vi "Read ADU Packet.vi"(8 "error in":errorcluster, 10 "protocol layer":refnum<class "Network Protocol.lvclass">, 11 "IP transmission data unit in":refnum<class "IP Data Unit.lvclass">) -> (0 "error out":errorcluster, 1 "modbus data unit":refnum<class "Modbus Data Unit.lvclass">, 2 "protocol layer out":refnum<class "Network Protocol.lvclass">, 3 "IP transmission data unit out":refnum<class "IP Data Unit.lvclass">, 5 "PDU Valid?":bool)   [LabVIEW 2013, in "IP Data Unit.lvclass"]
doc: "This uses the protocol layer to read a modbus packet off of the bus, wrapped in the IP transmission data unit."
uses:
  IP Data Unit.lvclass
  Modbus Data Unit/Modbus Data Unit.lvclass
  Network Protocol/Network Protocol.lvclass
  Transmission Data Unit.lvclass/Transmission Data Unit.ctl
  IP Data Unit.lvclass/IP Data Unit.ctl
  Modbus Data Unit/Modbus Data Unit.lvclass/Modbus Data Unit.ctl
  Modbus Data Unit/Unflatten to PDU.vi
  <vilib>/ErrorRing/Error Ring.xnode
  Transmission Data Unit.lvclass
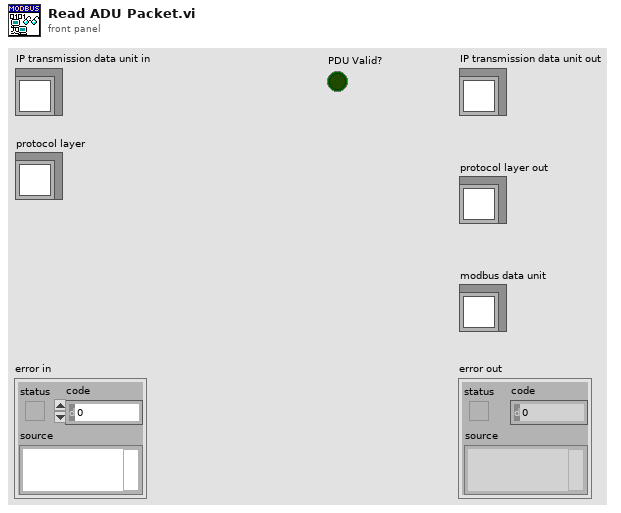
[diagram p1: front panel]
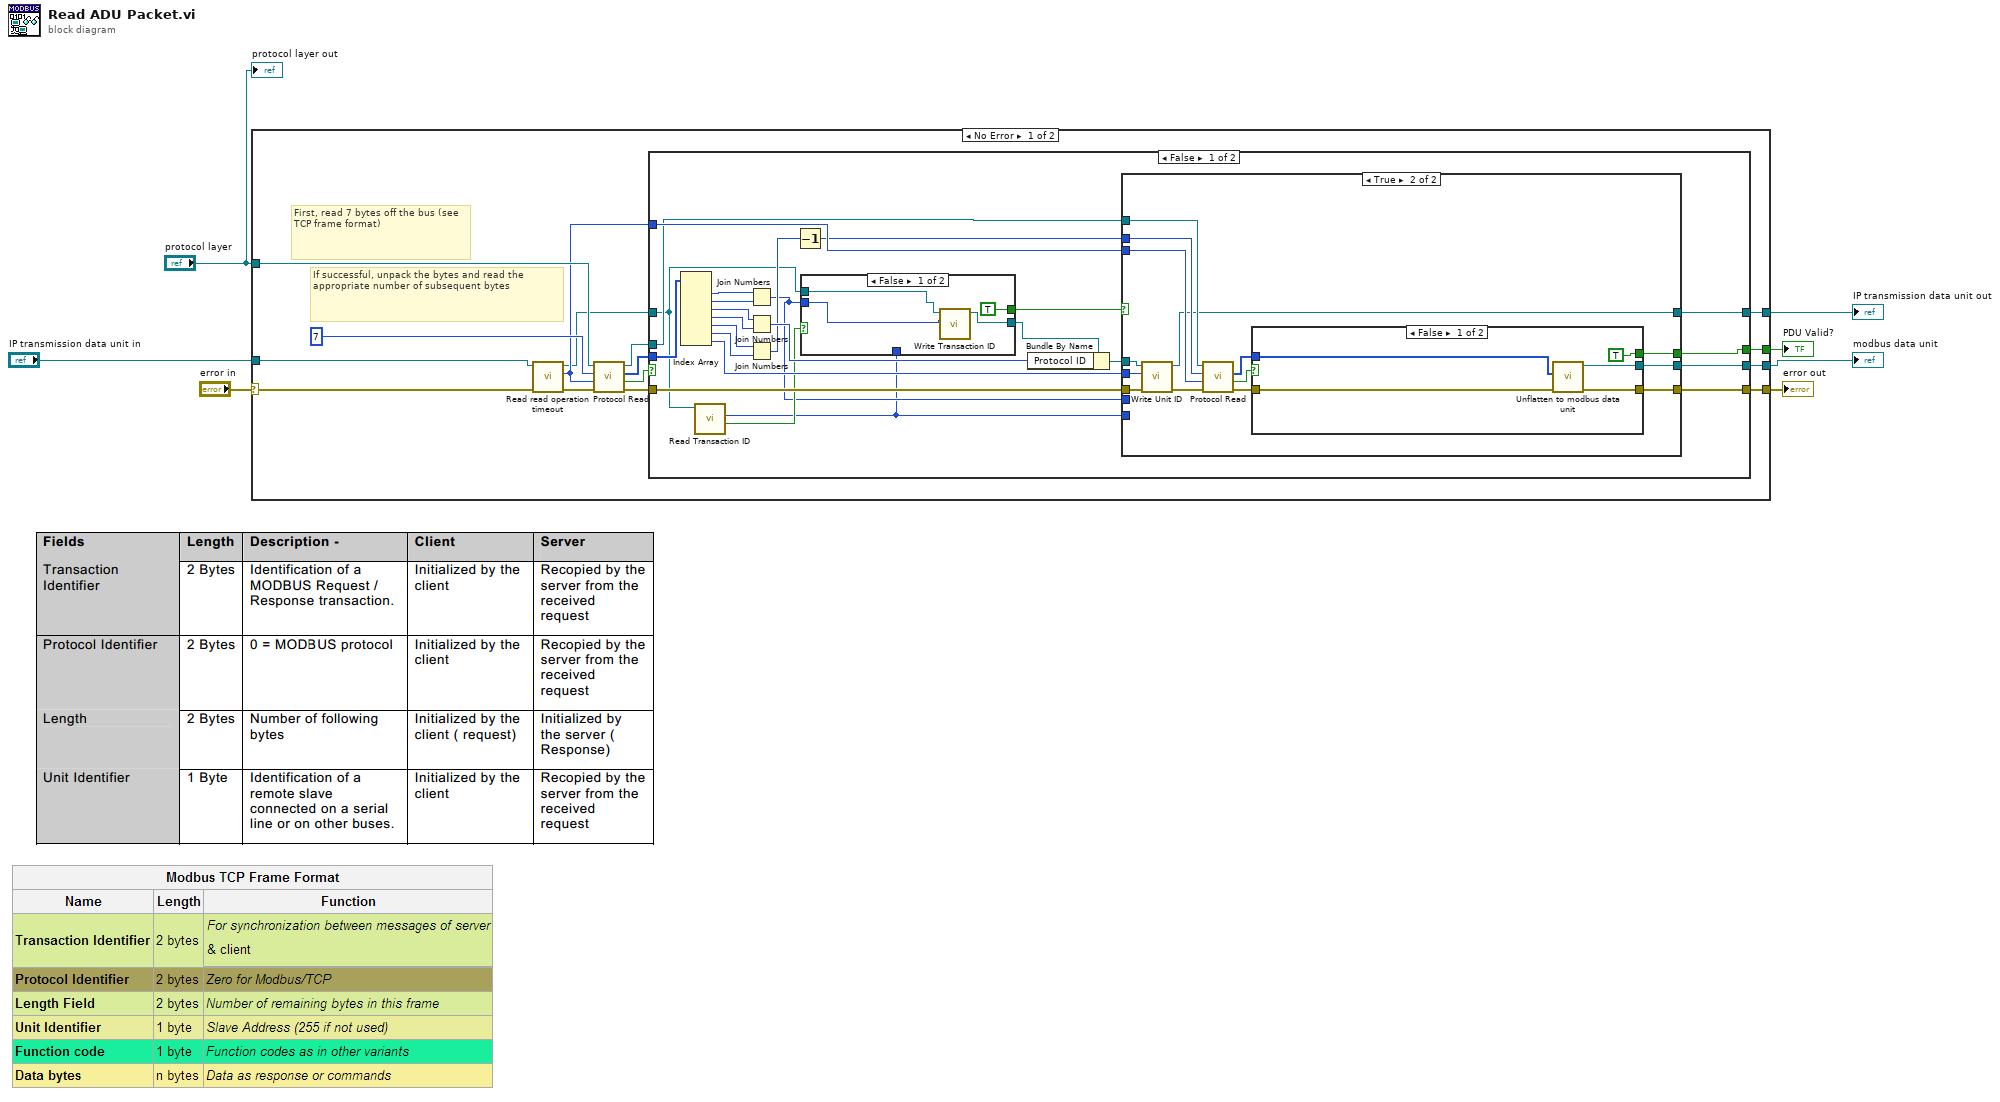
[diagram p0: block diagram]
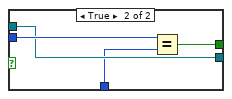
[diagram p2: hidden frame]
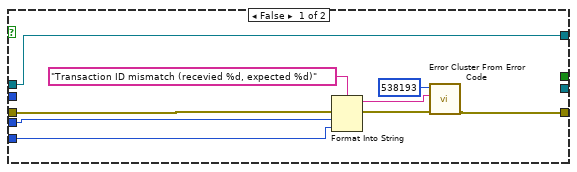
[diagram p3: hidden frame]
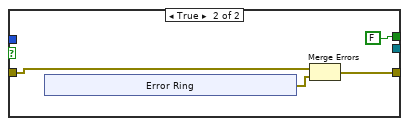
[diagram p4: hidden frame]
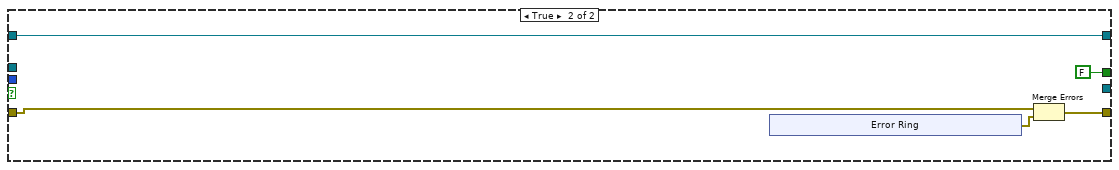
[diagram p5: hidden frame]
diagram:
  n1 = case shown="No Error" "error in" {
    selector: "error in" -> [w10 w102]
    tunnel: [w16 w102] -> w6
    tunnel: "IP transmission data unit in" -> [w12 w101]
    tunnel: [w19 w101] -> w4
    tunnel: "protocol layer" -> [w22 _]
    tunnel: [w15 _] -> w3
    tunnel: [w8 _] -> w1
    frame No Error {
      # "If successful, unpack the bytes and read the appropriate number of subsequent bytes"
      # "First, read 7 bytes off the bus (see TCP frame format)"
      n2 = call "Read read operation timeout.vi"("error in (no error)"=w10, "transmission data unit in"=w12) -> ("error out"=w9:errorcluster, "read operation timeout"=w13:i32, "transmission data unit out"=w11:refnum<class "IP Data Unit.lvclass">)  [unwired: 7 in]
      n3 = call-dynamic "Protocol Read.vi"("error in"=w9, "timeout"=w13, "bytes to read"=7 ("Bytes to Read"), "protocol layer in"=w22) -> ("error out"=w17:errorcluster, "timed out?"=w14:bool, "data"=w20:u8[], "protocol layer out"=w18:refnum<class "Network Protocol.lvclass">)  [unwired: 4 in]
      n4 = case shown="False" w14 {
        tunnel: w20 -> [w47 _]
        tunnel: w11 -> [w26 w96]
        tunnel: [w33 w96] -> w19
        tunnel: w18 -> [w29 _]
        tunnel: w13 -> [w38 _]
        tunnel: w17 -> [w27 w93]
        tunnel: [w36 w94] -> w16
        tunnel: [w35 _] -> w15
        tunnel: [w31 FALSE] -> w8
        frame False {
          n5 = Index Array(array=w47) -> (element #1=w45:u8, element #2=w46:u8, element #3=w44:u8, element #4=w43:u8, element #5=w40:u8, element #6=w41:u8, element #7=w32:u8)  [unwired: 7 in]
          n6 = call "Read Transaction ID.vi"("IP Data Unit in"=w26) -> ("Transaction ID set?"=w25:bool, "Transaction ID"=w23:u16)  [unwired: 8 in, 1 out]
          n7 = Join Numbers(hi=w45, lo=w46) -> ((hi.lo)=w24:u16)
          n8 = Join Numbers(hi=w44, lo=w43) -> ((hi.lo)=w42:u16)
          n9 = Join Numbers(hi=w40, lo=w41) -> ((hi.lo)=w39:u16)
          n10 = Decrement(x=w39) -> (x-1=w37:u16)
          n11 = case shown="False" w25 {
            tunnel: w26 -> [w50 w53]
            tunnel: w24 -> [w48 w55]
            tunnel: [TRUE w54] -> w30
            tunnel: [w49 w53] -> w28
            tunnel: w23 -> [_ w52]
            frame False {
              n12 = call "Write Transaction ID.vi"("Transaction ID"=w48, "IP Data Unit in"=w50) -> ("IP Data Unit out"=w49:refnum<class "IP Data Unit.lvclass">)  [unwired: 9 in]
            }
            frame True {
              n13 = Equal?(x=w55, y=w52) -> (x = y?=w54:bool)
            }
          }
          n14 = Bundle By Name(cluster=w28, "Protocol ID"=w42) -> (w34:refnum<class "IP Data Unit.lvclass">)
          n15 = case shown="True" w30 {
            tunnel: w29 -> [_ w78]
            tunnel: w38 -> [_ w77]
            tunnel: w37 -> [_ w76]
            tunnel: [w63 w74] -> w36
            tunnel: [_ w73] -> w35
            tunnel: w34 -> [w64 w70]
            tunnel: [w64 w69] -> w33
            tunnel: w27 -> [w61 w67]
            tunnel: w32 -> [_ w66]
            tunnel: [_ w65] -> w31
            tunnel: w24 -> [w57 _]
            tunnel: w23 -> [w56 _]
            frame False {
              n16 = Format Into String(format string="Transaction ID mismatch (recevied %d, expected %d)", error in=w61, w57, w56) -> (resulting string=w59:string, error out=w60:errorcluster)  [unwired: 1 in]
              n17 = call <vilib>:"Error Cluster From Error Code.vi"("error in (no error)"=w60, "error message (\"\")"=w59, "error code (0)"=538193) -> ("error out"=w63:errorcluster)  [unwired: 6 in]
            }
            frame True {
              n18 = call "Write Unit ID.vi"("error in"=w67, "unit ID"=w66, "transmission data unit in"=w70) -> ("error out"=w68:errorcluster, "transmission data unit out"=w69:refnum<class "IP Data Unit.lvclass">)  [unwired: 7 in]
              n19 = call-dynamic "Protocol Read.vi"("error in"=w68, "timeout"=w77, "bytes to read"=w76, "protocol layer in"=w78) -> ("error out"=w75:errorcluster, "timed out?"=w71:bool, "data"=w72:u8[])  [unwired: 4 in, 1 out]
              n20 = case shown="False" w71 {
                tunnel: w75 -> [w83 w86]
                tunnel: [w82 w87] -> w74
                tunnel: [w81 _] -> w73
                tunnel: w72 -> [w80 _]
                tunnel: [TRUE FALSE] -> w65
                frame False {
                  n21 = call "Unflatten to modbus data unit.vi"("error in"=w83, "modbus data unit data"=w80) -> ("error out"=w82:errorcluster, "modbus data unit out"=w81:refnum<class "Modbus Data Unit.lvclass">)  [unwired: 8 in]
                }
                frame True {
                  n22 = xnode "Error Ring"() -> ("error out"=w85:errorcluster)
                  n23 = Merge Errors(w86, w85) -> (w87:errorcluster)
                }
              }
            }
          }
        }
        frame True {
          n24 = xnode "Error Ring"() -> ("error out"=w95:errorcluster)
          n25 = Merge Errors(w93, w95) -> (w94:errorcluster)
        }
      }
    }
    frame Error {
    }
  }
  "error out" <- w6
  "IP transmission data unit out" <- w4
  "modbus data unit" <- w3
  "PDU Valid?" <- w1
  "protocol layer out" <- "protocol layer"
